vi "Pop Open.vi"(8 "error in (no error)":errorcluster, 11 "AD* in":refnum<class "NI_Robotics_AnytimeDStar.lvclass">) -> (0 "error out":errorcluster, 2 "node ref out":refnum<data-value>, 3 "AD* out":refnum<class "NI_Robotics_AnytimeDStar.lvclass">)   [LabVIEW 2017, in "NI_Robotics_AnytimeDStar.lvclass"]
uses:
  <vilib>/robotics/Navigation/Anytime D Star/NI_Robotics_AnytimeDStar.lvclass
  <vilib>/robotics/Navigation/shared/MapNode/AbstractDstarNode/NI_Robotics_AbstractDstarNode.lvclass
  <vilib>/robotics/Navigation/Anytime D Star/NI_Robotics_AnytimeDStar.lvclass/NI_Robotics_AnytimeDStar.ctl
  <vilib>/robotics/Navigation/shared/Priority Queue/NI_Robotics_Priority Queue.lvclass
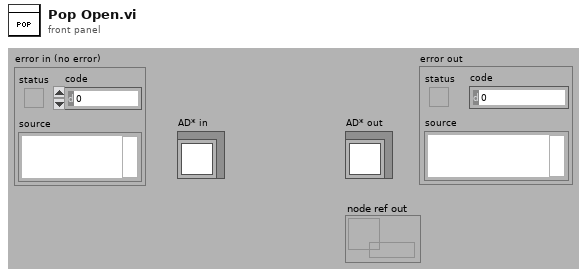
[diagram p1: front panel]
types:
  T1 = typedef "NI_Robotics_Priority Queue.lvclass/Open List Element.ctl" = cluster{"f":dbl, "g":dbl, "node Ref":refnum<data-value>}
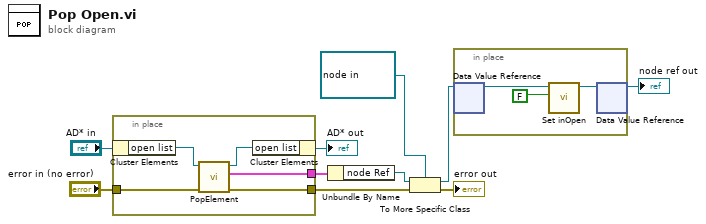
[diagram p0: block diagram]
diagram:
  n1 = in-place {
    in-place-border: [w15] -> w10
    in-place-border: "error in (no error)" -> [w12]
    in-place-border: [w11] -> w2
    n2 = in-place-cluster #1("AD* in") -> ("open list"=w14:refnum<class "NI_Robotics_Priority Queue.lvclass">)
    n3 = call <vilib>:"PopElement.vi"("error in (no error)"=w12, "Astar Open List in"=w14) -> ("error out"=w11:errorcluster, "open list element"=w15:T1, "Astar Open List out"=w13:refnum<class "NI_Robotics_Priority Queue.lvclass">)  [unwired: 6 in, 1 out]
    n4 = in-place-cluster #1("open list"=w13) -> (→"AD* out":refnum<class "NI_Robotics_AnytimeDStar.lvclass">)
  }
  n5 = Unbundle By Name(w10) -> ("node Ref"=w9:refnum<data-value>)
  n6 = To More Specific Class(target class=refnum<data-value> refnum ("node ref out"), reference=w9, error in=w2) -> (specific class reference=w8:refnum<data-value>, error out=→"error out":errorcluster)
  n7 = in-place {
    n8 = in-place-dvr #2(w8) -> (w17:refnum<class "NI_Robotics_AbstractDstarNode.lvclass">)  [unwired: 1 out]
    n9 = call <vilib>:"Set inOpen.vi"("inOpen"=FALSE, "AbstractDstarNode in"=w17) -> ("AbstractDstarNode out"=w16:refnum<class "NI_Robotics_AbstractDstarNode.lvclass">)  [unwired: 8 in, 1 out]
    n10 = in-place-dvr #2(w16) -> (→"node ref out":refnum<data-value>)  [unwired: 1 out]
  }
